vi "ControlDriveDistance.vi"(11 "Robot Motion Commands":T1) -> ()   [LabVIEW 2019]
uses:
  Controls/Robot Pivot Motion Commands.ctl
  Controls/Pivot Motor Commands.ctl
  Controls/Robot Drive Mode.ctl
  <vilib>/Rock Robotics/WPI/Utilities/WPI_GetSetVariantRefNum.vi
  <vilib>/addons/control/pid/pid.llb/PID (DBL Array).vi
  <vilib>/Rock Robotics/Network Tables/NT Write Numeric Array.vi
  <vilib>/addons/control/pid/NI_PID_pid.lvlib
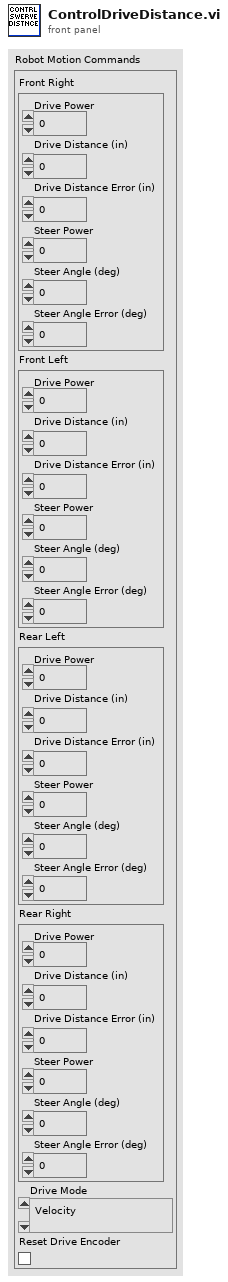
[diagram p1: front panel]
types:
  T1 = typedef "Robot Pivot Motion Commands.ctl" = cluster{"Front Right":T2, "Front Left":T2, "Rear Left":T2, "Rear Right":T2, "Drive Mode":T3, "Reset Drive Encoder":bool}
  T2 = typedef "Pivot Motor Commands.ctl" = cluster{"Drive Power":dbl, "Drive Distance (in)":dbl, "Drive Distance Error (in)":dbl, "Steer Power":dbl, "Steer Angle (deg)":dbl, "Steer Angle Error (deg)":dbl}
  T3 = typedef "Robot Drive Mode.ctl" = enum16{"Velocity", "Distance"}
  T4 = cluster{"proportional gain (Kc)":dbl, "integral time (Ti, min)":dbl, "derivative time (Td, min)":dbl}
  T5 = cluster{"proportional gain (Kc)":dbl, "integral time (Ti, min)":dbl, "derivative time (Td, min)":dbl}[]
  T6 = typedef "WPI_RobotDriveDevRef.ctl" = cluster{"DevStatus":errorcluster, "Motors[]":T7[], "Square Inputs":bool, "Max Output":dbl}
  T7 = typedef "WPI_MotorControlDeviceRef.ctl" = cluster{"DeviceStatus":errorcluster, "Type":T8, "PWM":cluster{"PWM Channel":T9, "DeadBand":T10}, "CAN":cluster{"Device Number":u8, "SetOutput VI Ref":variant, "GetOutput VI Ref":variant, "Enable VI Ref":variant, "Disable VI Ref":variant, "Data":variant}, "Invert":bool, "DIO PWM":cluster{"PWM \"Enable\" Channel":T9, "DIOChannel":T11, "PWM Rate":dbl}}
  T8 = typedef "WPI_MotorControlType.ctl" = enum16{"PWM", "CAN", "DIO PWM"}
  T9 = typedef "FPGA_DIOPWMChannel.ctl" = enum8{"PWM 0", "PWM 1", "PWM 2", "PWM 3", "PWM 4", "PWM 5", "PWM 6", "PWM 7", "PWM 8", "PWM 9", "PWM MXP 0", "PWM MXP 1", "PWM MXP 2", "PWM MXP 3", "PWM MXP 4", "PWM MXP 5", "PWM MXP 6", "PWM MXP 7", "PWM MXP 8", "PWM MXP 9", "Invalid"}
  T10 = typedef "WPI_PWMDeadband.ctl" = cluster{"Name":string, "maxPositivePwm":i32, "minPositivePwm":i32, "centerPwm":i32, "maxNegativePwm":i32, "minNegativePwm":i32, "angularRange":u16}
  T11 = typedef "FPGA_DIOChannel.ctl" = enum8{"DIO 0", "DIO 1", "DIO 2", "DIO 3", "DIO 4", "DIO 5", "DIO 6", "DIO 7", "DIO 8", "DIO 9", "DIO MXP 0", "DIO MXP 1", "DIO MXP 2", "DIO MXP 3", "DIO MXP 4", "DIO MXP 5", "DIO MXP 6", "DIO MXP 7", "DIO MXP 8", "DIO MXP 9", "DIO MXP 10", "DIO MXP 11", "DIO MXP 12", "DIO MXP 13", "DIO MXP 14", "DIO MXP 15", "SPI Port CS1", "SPI Port CS2", "SPI Port CS3", "SPI Port MISO", "SPI Port MOSI", "Invalid"}
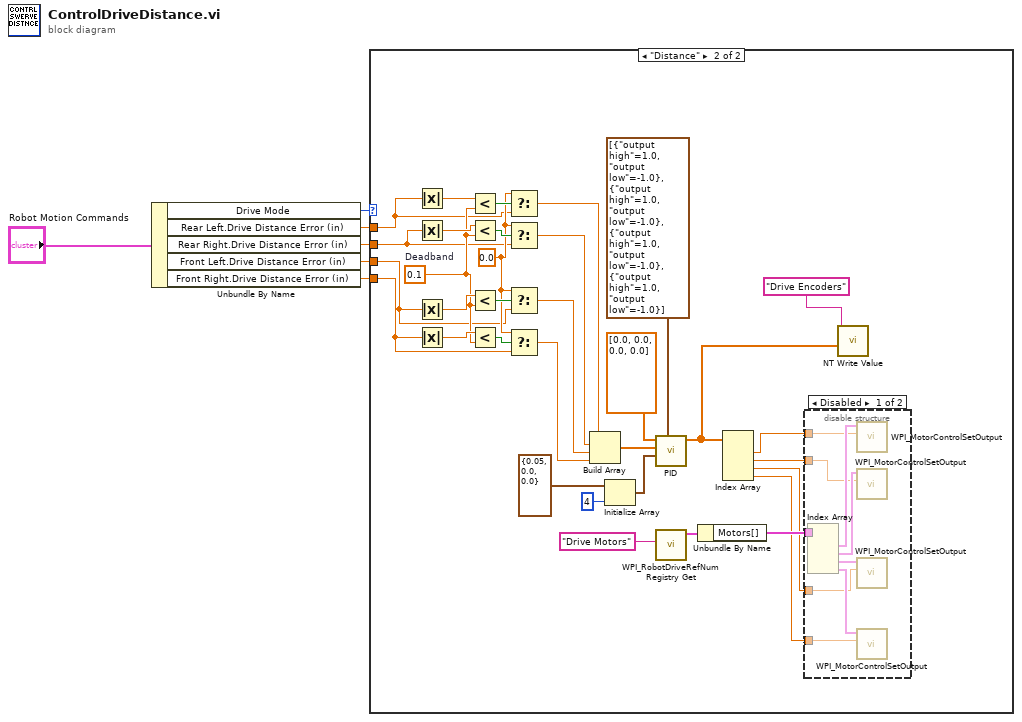
[diagram p0: block diagram]
diagram:
  n1 = Unbundle By Name("Robot Motion Commands") -> ("Drive Mode"=w1:T3, "Rear Left.Drive Distance Error (in)"=w5:dbl, "Rear Right.Drive Distance Error (in)"=w4:dbl, "Front Left.Drive Distance Error (in)"=w2:dbl, "Front Right.Drive Distance Error (in)"=w3:dbl)
  n2 = case shown="\"Distance\"" w1 {
    tunnel: w5 -> [_ w12]
    tunnel: w4 -> [_ w11]
    tunnel: w3 -> [_ w10]
    tunnel: w2 -> [_ w9]
    frame "Velocity", Default {
      # "do nothing in velocity mode"
    }
    frame "Distance" {
      w18 = 0.0
      w13 = 0.1  # Deadband
      n3 = Absolute Value(x=w12) -> (abs(x)=w20:dbl)
      n4 = Absolute Value(x=w11) -> (abs(x)=w22:dbl)
      n5 = Absolute Value(x=w9) -> (abs(x)=w24:dbl)
      n6 = Absolute Value(x=w10) -> (abs(x)=w26:dbl)
      n7 = Less?(x=w20, y=w13) -> (x < y?=w19:bool)
      n8 = Less?(x=w22, y=w13) -> (x < y?=w21:bool)
      n9 = Less?(x=w24, y=w13) -> (x < y?=w23:bool)
      n10 = Less?(x=w26, y=w13) -> (x < y?=w25:bool)
      n11 = Select(t=w18, s=w19, f=w12) -> (s? t:f=w17:dbl)
      n12 = Select(t=w18, s=w21, f=w11) -> (s? t:f=w16:dbl)
      n13 = Select(t=w18, s=w23, f=w9) -> (s? t:f=w15:dbl)
      n14 = Select(t=w18, s=w25, f=w10) -> (s? t:f=w14:dbl)
      n15 = Build Array(w17, w16, w15, w14) -> (w32:dbl[])
      n16 = Initialize Array(T4 {"proportional gain (Kc)"=0.05, "integral time (Ti, min)"=0.0, "derivative time (Td, min)"=0.0} ("PID gains"), 4 ("dimension size")) -> (w33:T5)
      n17 = call-poly <vilib>:"PID.vi"("output range"=cluster{"output high":dbl, "output low":dbl}[] [{"output high"=1.0, "output low"=-1.0}, {"output high"=1.0, "output low"=-1.0}, {"output high"=1.0, "output low"=-1.0}, {"output high"=1.0, "output low"=-1.0}], "PID gains"=w33, "process variable"=w32, "setpoint"=dbl[] [0.0, 0.0, 0.0, 0.0]) -> ("output"=w8:dbl[])  [unwired: 6 in, 1 out]
      n18 = call <vilib>:"WPI_RobotDriveRefNum Registry Get.vi"("refnum name"="Drive Motors") -> ("RobotDriveDevRef"=w38:T6)  [unwired: 9 in, 1 out]
      n19 = Unbundle By Name(w38) -> ("Motors[]"=w31:T7[])
      n20 = Index Array(array=w8) -> (element #1=w30:dbl, element #2=w29:dbl, element #3=w28:dbl, element #4=w27:dbl)  [unwired: 4 in]
      n21 = disable-structure shown="Disabled" {
        disable-tunnel: w31 -> [w48 _]
        disable-tunnel: w30 -> [w43 _]
        disable-tunnel: w29 -> [w42 _]
        disable-tunnel: w28 -> [w41 _]
        disable-tunnel: w27 -> [w40 _]
        frame Disabled {
          n22 = Index Array(array=w48) -> (element #1=w47:T7, element #2=w46:T7, element #3=w45:T7, element #4=w44:T7)  [unwired: 4 in]
          n23 = call <vilib>:"WPI_MotorControlSetOutput.vi"("Output"=w43, "MotorControlDevRef"=w47) -> ()  [unwired: 7 in, 3 out]
          n24 = call <vilib>:"WPI_MotorControlSetOutput.vi"("Output"=w42, "MotorControlDevRef"=w46) -> ()  [unwired: 7 in, 3 out]
          n25 = call <vilib>:"WPI_MotorControlSetOutput.vi"("Output"=w41, "MotorControlDevRef"=w45) -> ()  [unwired: 7 in, 3 out]
          n26 = call <vilib>:"WPI_MotorControlSetOutput.vi"("Output"=w40, "MotorControlDevRef"=w44) -> ()  [unwired: 7 in, 3 out]
        }
        frame Enabled {
        }
      }
      n27 = call-poly <vilib>:"NT Write Value.vi"("Numeric Array"=w8, "Name"="Drive Encoders") -> ()  [unwired: 9 in, 1 out]
    }
  }
